vi "Unpack for gRPC.vi"(8 "error in":errorcluster, 9 "configuration / results":enum16{"Configuration", "Results"}(ring), 10 "any":T1, 11 "measurement customizations in":refnum<class "Measurement Plugin.lvclass">) -> (0 "error out":errorcluster, 2 "data value":variant, 3 "measurement customizations out":refnum<class "Measurement Plugin.lvclass">)   [LabVIEW 2024, in "OneShot-PureTone.lvlib" / "Measurement Plugin.lvclass"]
uses:
  Measurement Plugin.lvclass
  Measurement Plugin.lvclass/Measurement Plugin.ctl
  Measurement Configuration.ctl
  OneShot-PureTone.lvlib
  Measurement Results.ctl
  3ecd018e-d556-4cbc-bc60-c4ba57204520.vi
  a521b266-ce99-437c-923d-067dcf1e07fd.vi
  <vilib>/Plug-In SDKs/Measurements/Measurement Plugin Service/Measurement Plugin Service.lvclass
  <vilib>/gRPC/LabVIEW gRPC Library/Shared/Any.ctl
  <vilib>/gRPC/LabVIEW gRPC Library/grpc-lvsupport-release.lvlib
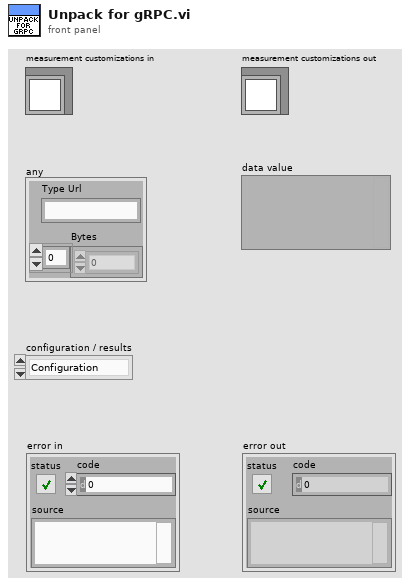
[diagram p1: front panel]
types:
  T1 = typedef "grpc-lvsupport-release.lvlib/Any.ctl" = cluster{"Type Url":string, "Bytes":u8[]}
  T2 = typedef "grpc-lvsupport-release.lvlib/grpcId.ctl" = u64
  T3 = typedef "OneShot-PureTone.lvlib/Measurement Configuration.ctl" = cluster{"THD maximum harmonic":i32, "measurement duration (s)":dbl, "measurement cycles":dbl, "band start (Hz)":dbl, "band stop (Hz)":dbl, "ramp up (s)":dbl, "ramp down (s)":dbl, "settle time (s)":dbl, "settle cycles":dbl, "AI range":dbl, "AO range":dbl, "output channel":string, "input channel":string, "frequency (Hz)":dbl, "amplitude":dbl, "sample rate (Hz)":dbl}
  T4 = typedef "OneShot-PureTone.lvlib/Measurement Results.ctl" = cluster{"band start (Hz) out":dbl, "band stop (Hz) out":dbl, "detected frequency (Hz)":dbl, "detected amplitude":dbl, "acquired response":dbl[], "measurement subset":dbl[], "acquired response t0":dbl, "acquired response dt":dbl, "measurement subset t0":dbl, "measurement subset dt":dbl, "error":bool, "error code":i32, "error source":string, "THD maximum harmonic out":i32}
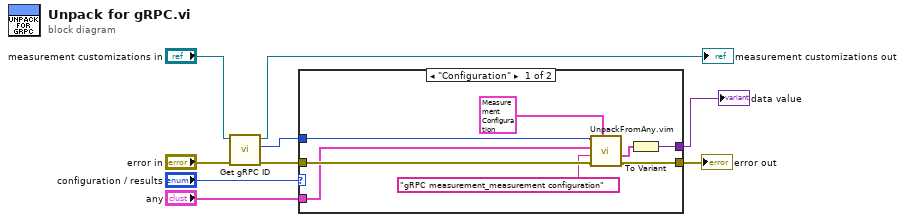
[diagram p0: block diagram]
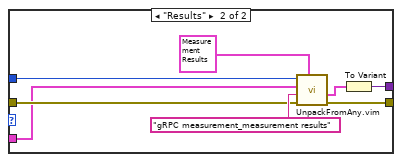
[diagram p2: hidden frame]
diagram:
  n1 = call <vilib>:"Get gRPC ID.vi"("error in"="error in", "measurement plugin service in"="measurement customizations in") -> ("error out"=w6:errorcluster, "gRPC ID"=w3:T2, "measurement plugin service out"=→"measurement customizations out":refnum<class "Measurement Plugin.lvclass">)  [unwired: 7 in]
  n2 = case shown="\"Configuration\"" "configuration / results" {
    tunnel: w6 -> [w15 w19]
    tunnel: "any" -> [w10 w18]
    tunnel: w3 -> [w12 w22]
    tunnel: [w16 w23] -> w9
    tunnel: [w17 w25] -> w1
    frame "Configuration" {
      n3 = call "UnpackFromAny.vim"("Data Type"=T3 {"THD maximum harmonic"=-32, "measurement duration (s)"=32.0, "measurement cycles"=1.0, "band start (Hz)"=1.0, "band stop (Hz)"=20000.0, "ramp up (s)"=0.02, "ramp down (s)"=0.01, "settle time (s)"=0.01, "settle cycles"=10.0, "AI range"=3.0, "AO range"=3.5, "output channel"="Lorem ipsum dolor sit", "input channel"="Dev1/ai0", "frequency (Hz)"=1000.0, "amplitude"=1.0, "sample rate (Hz)"=51200.0} ("Measurement Configuration"), "error in"=w15, "Message Type"="gRPC measurement_measurement configuration", "Any"=w10, "gRPCid in"=w12) -> ("error out"=w16:errorcluster, "Unpacked Value"=w14:T3)  [unwired: 4 in, 1 out]
      n4 = To Variant(anything=w14) -> (Variant=w17:variant)
    }
    frame "Results" {
      n5 = call "UnpackFromAny.vim"("Data Type"=T4 {"band start (Hz) out"=0.0, "band stop (Hz) out"=0.0, "detected frequency (Hz)"=0.0, "detected amplitude"=0.0, "acquired response"=[], "measurement subset"=[], "acquired response t0"=0.0, "acquired response dt"=0.0, "measurement subset t0"=0.0, "measurement subset dt"=0.0, "error"=FALSE, "error code"=0, "error source"="Empty", "THD maximum harmonic out"=9} ("Measurement Results"), "error in"=w19, "Message Type"="gRPC measurement_measurement results", "Any"=w18, "gRPCid in"=w22) -> ("error out"=w23:errorcluster, "Unpacked Value"=w24:T4)  [unwired: 4 in, 1 out]
      n6 = To Variant(anything=w24) -> (Variant=w25:variant)
    }
  }
  "error out" <- w9
  "data value" <- w1
